vi "LoadImage_Names_Array.vi"(8 "First Image":i32, 9 "Load in PCO Format":bool, 10 "Load Array":bool, 11 "Sample Image":path) -> (0 "Image Filenames":string[](array[string]), 1 "Paths":path[](array[path]), 3 "Film length":i32)   [LabVIEW 2010]
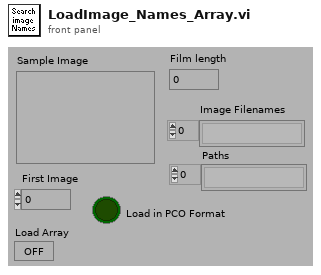
[diagram p1: front panel]
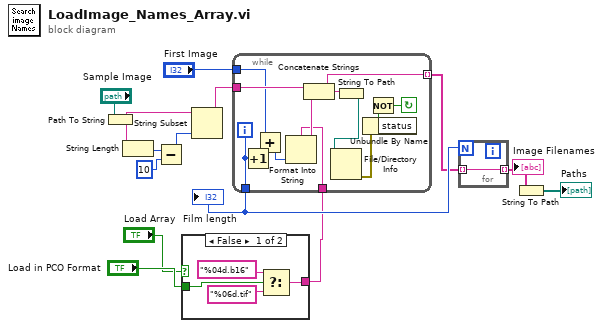
[diagram p0: block diagram]
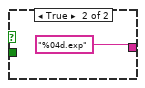
[diagram p2: hidden frame]
diagram:
  n1 = Path To String(path="Sample Image") -> (string=w9:string)
  n2 = String Length(string=w9) -> (length=w12:i32)
  n3 = Subtract(x=w12, y=10) -> (x-y=w10:i32)
  n4 = case shown="False" "Load Array" {
    tunnel: [w18 "%04d.exp" ("t")] -> w3
    tunnel: "Load in PCO Format" -> [w17 _]
    frame False {
      n5 = Select(t="%04d.b16", s=w17, f="%06d.tif" ("Format String")) -> (s? t:f=w18:string)
    }
    frame True {
    }
  }
  n6 = String Subset(string=w9, length (rest)=w10) -> (substring=w8:string)  [unwired: 1 in]
  n7 = while {
    tunnel: "First Image" -> [w23]
    tunnel: [w26] -> w7 mode=indexing
    tunnel: w8 -> [w28]
    tunnel: [w29] -> w14
    tunnel: w3 -> [w20]
    i -> [w29]
    stop <- w30 continue-if-true
    n8 = Increment(x=w29) -> (x+1=w25:i32)
    n9 = Add(x=w23, y=w25) -> (x+y=w24:i32)
    n10 = Format Into String(format string=w20, w24) -> (resulting string=w27:string)  [unwired: 2 in, 1 out]
    n11 = Concatenate Strings(w28, w27) -> (w26:string)
    n12 = String To Path(string=w26) -> (path=w21:path)
    n13 = File/Directory Info(path=w21) -> (error out=w22:errorcluster)  [unwired: 1 in, 6 out]
    n14 = Unbundle By Name(w22) -> ("status"=w31:bool)
    n15 = Not(x=w31) -> (.not. x?=w30:bool)
  }
  "Film length" <- w14
  n16 = for {
    N: w14 -> [_]
    tunnel: [w32] -> w6 mode=indexing
    tunnel: w7 -> [w32] mode=indexing
  }
  "Image Filenames" <- w6
  n17 = String To Path(string=w6) -> (path=→"Paths":path[])
